vi "Method One Numeric Argument.vi"(8 "error in (no error)":errorcluster, 10 "Numeric":dbl, 11 "Test Interface Mock In":refnum<class "Test Interface Responsive Mock.lvclass">) -> (0 "error out":errorcluster, 3 "Test Interface Mock Out":refnum<class "Test Interface Responsive Mock.lvclass">)   [LabVIEW 2020, in "Test Interface Responsive Mock.lvclass"]
uses:
  Test Interface Responsive Mock.lvclass
  C:/git/astemes-lmock/source/Framework/Responsive Mock/Responsive Mock.lvclass
  source/Framework/Responsive Mock/Responsive Mock.lvclass/Responsive Mock.ctl
  source/Framework/Parametric VI Call/Parametric VI Call.lvclass
  C:/git/astemes-lmock/source/Core/VI Call/VI Call.lvclass
  source/Framework/Parametric VI Call/Create.vi
  source/Core/Expectation/Expectation.lvclass
  source/Framework/Responsive Mock/Responsive Mock.lvclass
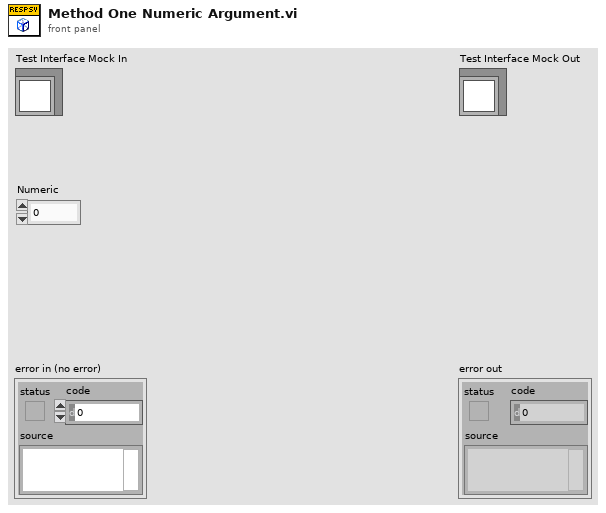
[diagram p1: front panel]
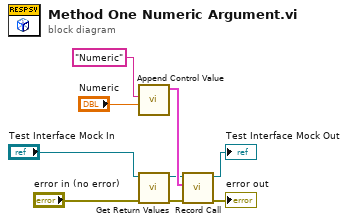
[diagram p0: block diagram]
diagram:
  n1 = call "Append Control Value.vi"("Variant Data"="Numeric", "Name"="Numeric") -> ("Control Values"=w4:cluster{"Name":string, "Variant Data":variant}[])  [unwired: 9 in]
  n2 = call "Get Return Values.vi"("error in (no error)"="error in (no error)", "Mock In"="Test Interface Mock In") -> ("error out"=w1:errorcluster, "Mock Out"=w2:refnum<class "Test Interface Responsive Mock.lvclass">)  [unwired: 7 in, 1 out]
  n3 = call "Record Call.vi"("error in (no error)"=w1, "Control Values"=w4, "Mock In"=w2) -> ("error out"=→"error out":errorcluster, "Mock Out"=→"Test Interface Mock Out":refnum<class "Test Interface Responsive Mock.lvclass">)  [unwired: 7 in]
